vi "Practica_2_Area del Triangulo.vi"() -> ()   [LabVIEW 2022 SP3]
panel:
  out "Area (cm^2)":dbl
  in  "Alturaa (cm)":dbl
  in  "Base (cm)":dbl
  # "AREA DEL TRIANGULO"
  # "ALTURA"
  # "BASE"
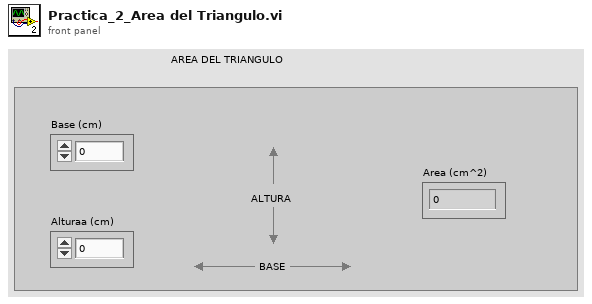
[diagram p1: front panel]
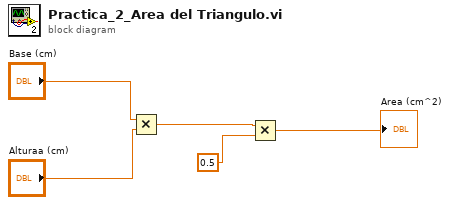
[diagram p0: block diagram]
diagram:
  n1 = Multiply(x="Base (cm)", y="Alturaa (cm)") -> (x*y=w3:dbl)
  n2 = Multiply(x=w3, y=0.5) -> (x*y=→"Area (cm^2)":dbl)
